vi "字幕.vi"() -> ()   [LabVIEW 2018]
panel:
  in  "开始":bool
  out "大小":i32
  out "数值":i32=760
  in  "停止":bool
  out "显示框(有时需等待)":bool[][](array[boolean])
  in  "字符串":string="祝你开心快乐"
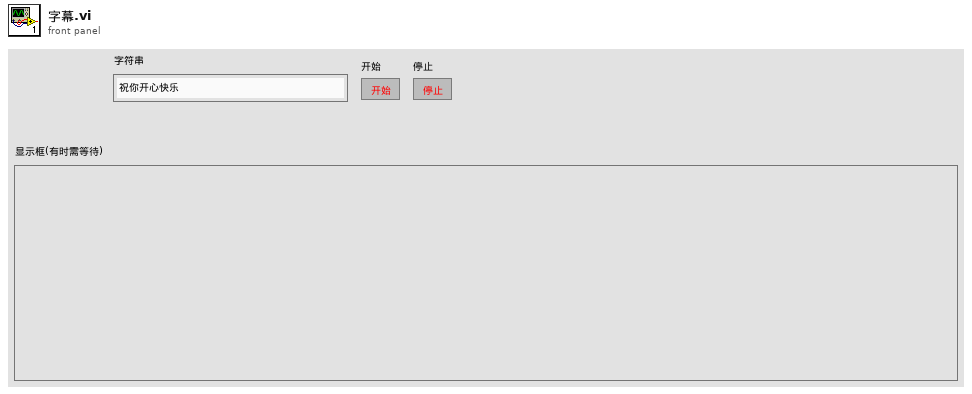
[diagram p1: front panel]
types:
  T1 = typedef "imagedata.ctl" = cluster{"image type":i32, "image depth":i32, "image":u8[], "mask":u8[], "colors":u32[], "Rectangle":cluster{"left":i16, "top":i16, "right":i16, "bottom":i16}}
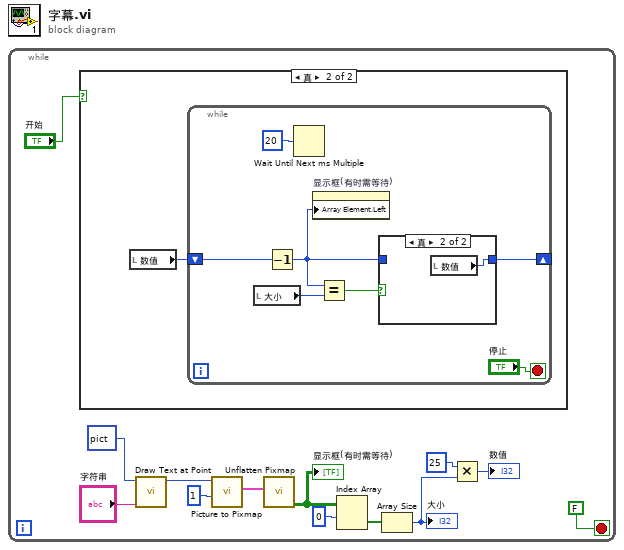
[diagram p0: block diagram]
diagram:
  n1 = while {
    stop <- FALSE stop-if-true
    n2 = case shown="真" "开始" {
      frame False {
      }
      frame True {
        n3 = local read "数值"() -> (w14:i32)
        n4 = while {
          shift-right: [w17] -> _
          shift-left: w14 -> [w18]
          stop <- "停止" stop-if-true
          n5 = local read "大小"() -> (w15:i32)
          n6 = Decrement(x=w18) -> (x-1=w16:i32)
          n7 = Wait Until Next ms Multiple(millisecond multiple=u32 20 ("毫秒倍数")) -> ()  [unwired: 1 out]
          n8 = property on="显示框(有时需等待)" class="Arr (严格)"("Array Element.Left"=w16) -> ()  [unwired: 2 in, 2 out]
          n9 = Equal?(x=w16, y=w15) -> (x = y?=w19:bool)
          n10 = case shown="真" w19 {
            tunnel: [w22 w23] -> w17
            tunnel: w16 -> [w22 _]
            frame False {
            }
            frame True {
              n11 = local read "数值"() -> (w23:i32)
            }
          }
        }
      }
    }
    n12 = call <vilib>:"Draw Text at Point.vi"("text"="字符串", "picture"=picture data[5B]) -> ("new picture"=w12:picture)  [unwired: 8 in, 1 out]
    n13 = call <vilib>:"Picture to Pixmap.vi"("depth"=1, "picture"=w12) -> ("image data"=w13:T1)  [unwired: 8 in, 1 out]
    n14 = call <vilib>:"Unflatten Pixmap.vi"("image data"=w13) -> ("1-bit pixmap"=w8:bool[][])  [unwired: 4 in, 6 out]
    "显示框(有时需等待)" <- w8
    n15 = Index Array(array=w8, index (row)=0 ("索引 (行)")) -> (element=w6:bool[])  [unwired: 1 in]
    n16 = Array Size(array=w6) -> (size(s)=w5:i32)
    "大小" <- w5
    n17 = Multiply(x=25, y=w5) -> (x*y=→"数值":i32)
  }
